vi "HRTF-Devices Dialog (TDT).vi"(1 "Path":path) -> (8 "Canceled?":bool)   [LabVIEW 2015]
uses:
  Utility VIs/Controls/KTable/KTable.xctl
  Typedefs/HRTF-Hardware Config (TDT).ctl
  PXI DAQ VIs/TDT VIs/Typedefs/TDT-Output source.ctl
  PXI DAQ VIs/TDT VIs/Typedefs/TDT-Device ID.ctl
  PXI DAQ VIs/TDT VIs/TDT-Globals.vi
panel:
  in  "InputTable":u16(xcontrol)
  in  "OutputTable":u16(xcontrol)
  out "Image":enum32{"None", "RX6", "RZ5", "RZ6"}(tab)
  in  "Run on":u16(ring) items=["RX6", "RZ5", "RZ6"]
  out "exit signal":bool
  in  "Cancel":bool
  in  "OK":bool
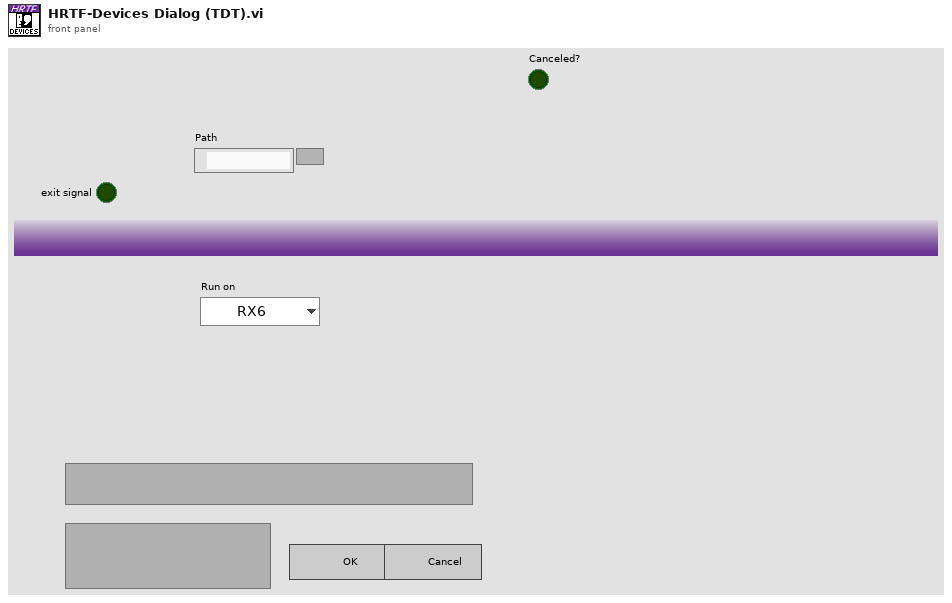
[diagram p1: front panel]
types:
  T1 = typedef "HRTF-Hardware Config (TDT).ctl" = cluster{"Output":T2, "Speaker":cluster{"Channel":i32, "Primary mux":i32, "Secondary mux":i32}, "Right mic":i32, "Left mic":i32}
  T2 = typedef "TDT-Output source.ctl" = cluster{"Device":T3, "Num":i32}
  T3 = typedef "TDT-Device ID.ctl" = enum16{"None", "PA5", "RP2", "RL2", "RA16", "RV8", "RX5", "RX6", "RX7", "RX8", "RZ2", "RZ5", "RZ6"}
  T4 = cluster{string, "Channel":i32, "Primary mux":i32, "Secondary mux":i32}
  T5 = cluster{string, "Channel":i32, "Primary mux":i32, "Secondary mux":i32}[]
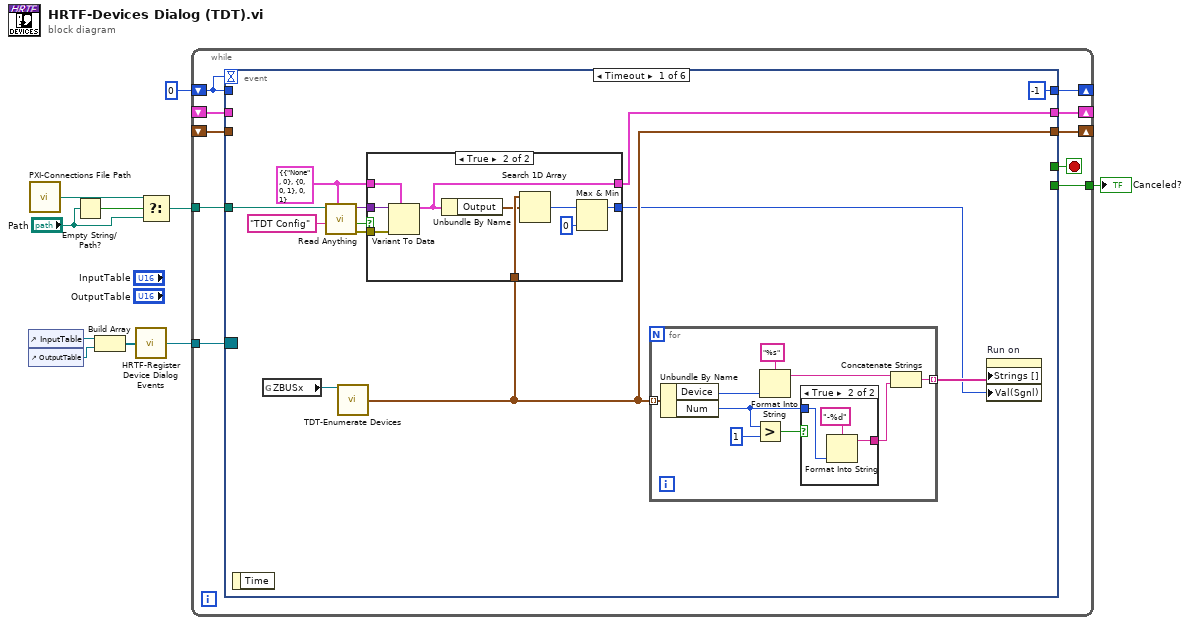
[diagram p0: block diagram]
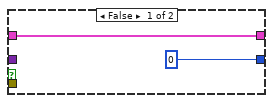
[diagram p2: hidden frame]
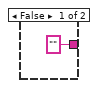
[diagram p3: hidden frame]
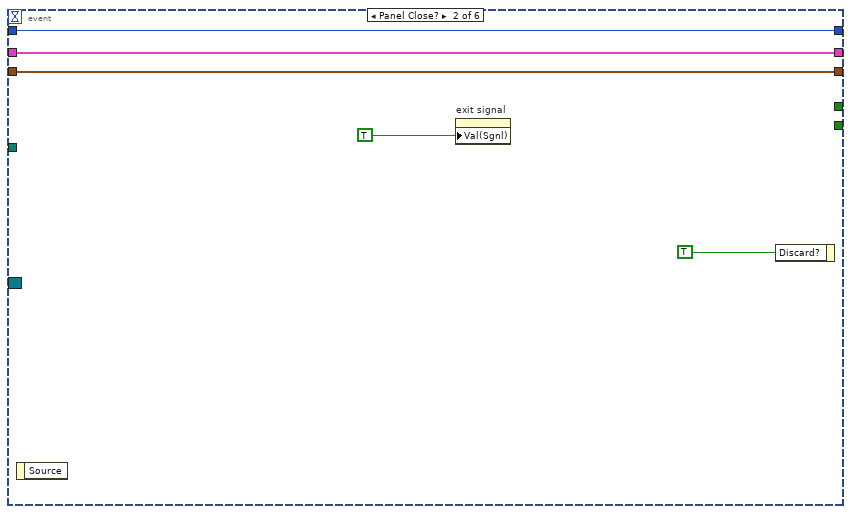
[diagram p4: hidden frame]
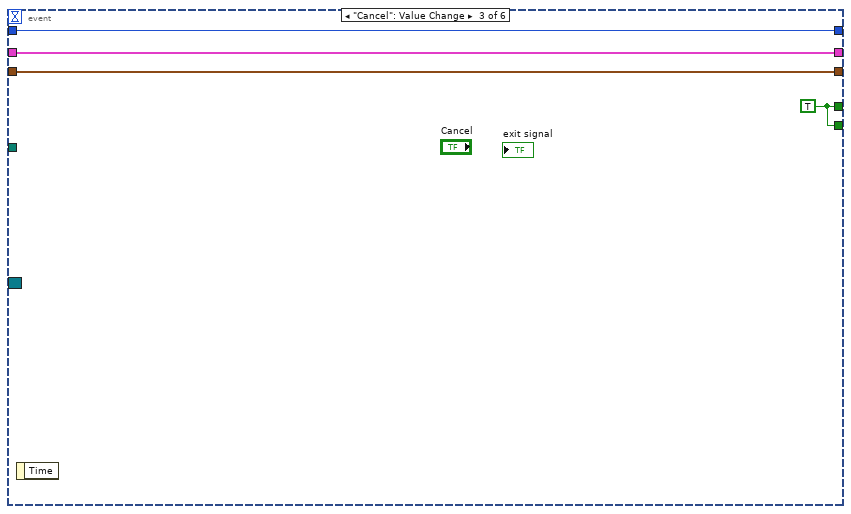
[diagram p5: hidden frame]
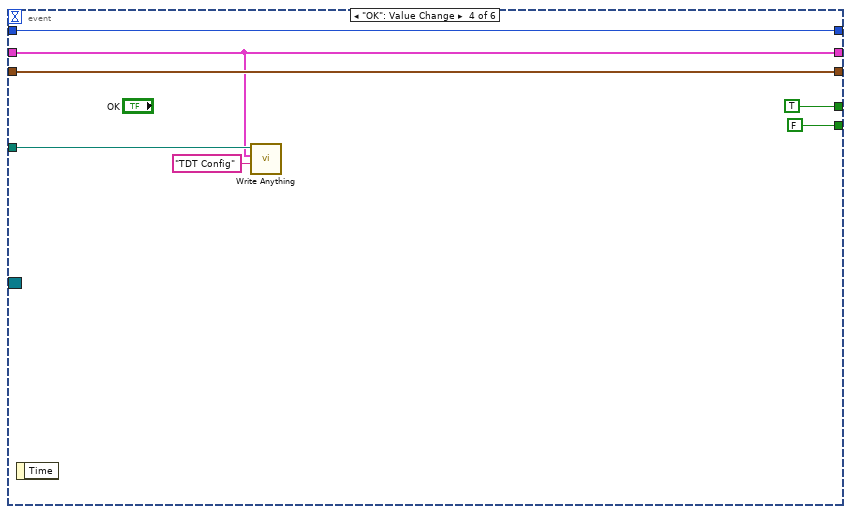
[diagram p6: hidden frame]
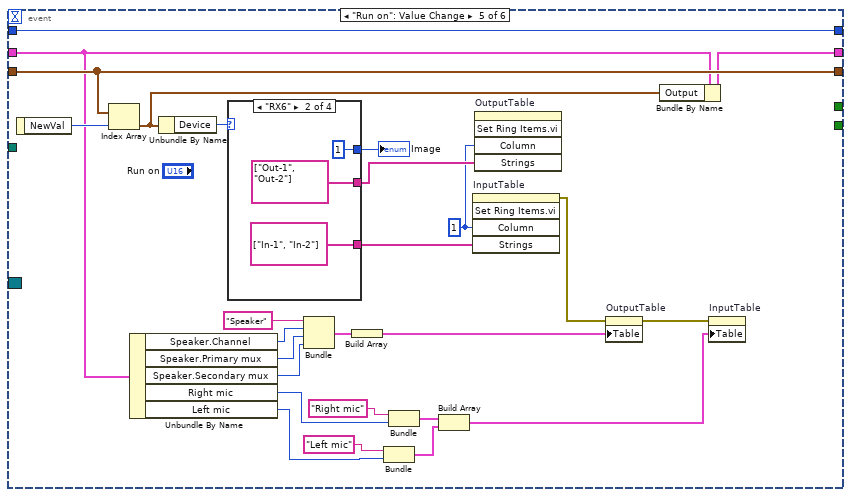
[diagram p7: hidden frame]
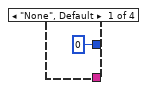
[diagram p8: hidden frame]
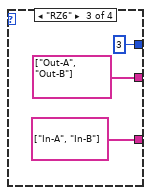
[diagram p9: hidden frame]
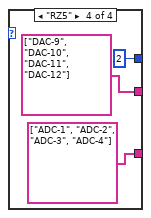
[diagram p10: hidden frame]
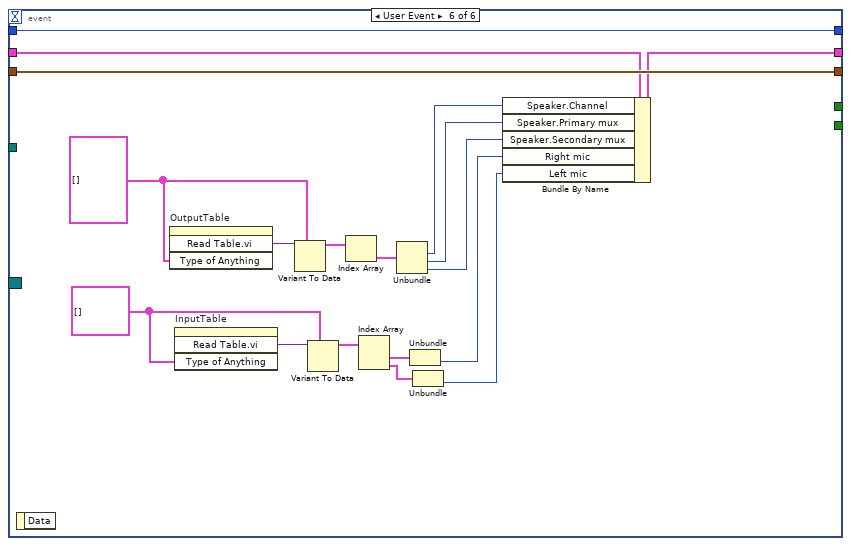
[diagram p11: hidden frame]
diagram:
  n1 = control-ref of="InputTable"() -> (w4:refnum<vi>)
  n2 = control-ref of="OutputTable"() -> (w3:refnum<vi>)
  n3 = call "PXI-Connections File Path.vi"() -> ("Path"=w7:path)  [unwired: 1 in]
  n4 = Empty String/Path?(string/path="Path") -> (empty?=w8:bool)
  n5 = Build Array(w4, w3) -> (w2:refnum<vi>[])
  n6 = call "HRTF-Register Device Dialog Events.vi"("Refs"=w2) -> ("Event Registration Refnum"=w1:refnum<event-registration>)  [unwired: 13 in, 1 out]
  n7 = Select(t=w7, s=w8, f="Path") -> (s? t:f=w5:path)
  n8 = while {
    shift-right: [w20] -> _
    shift-left: 0 -> [w17]
    tunnel: [w18] -> w9
    shift-right: [w16] -> _
    shift-left: _ -> [w15]
    tunnel: w5 -> [w14]
    shift-right: [w13] -> _
    shift-left: _ -> [w12]
    tunnel: w1 -> [w11]
    stop <- w19 stop-if-true
    n9 = event shown="[0] Timeout" {
      selector: w11 -> [_ _ _ _ _ _]
      dyn-events: _ -> [_ _ _ _ _ _]
      timeout: w17 -> [_ _ _ _ _ _]
      tunnel: [-1 w61 w64 w70 w98 w126] -> w20
      tunnel: [_ _ w65 TRUE _ _] -> w19
      tunnel: [_ _ w65 FALSE _ _] -> w18
      tunnel: w17 -> [_ w61 w64 w70 w98 w126]
      tunnel: [w25 w58 w63 w69 w97 w125] -> w16
      tunnel: w15 -> [_ w58 w63 w69 w97 w125]
      tunnel: w14 -> [w30 _ _ w68 _ _]
      tunnel: [w21 w57 w62 w67 w74 w119] -> w13
      tunnel: w12 -> [_ w57 w62 w67 w90 w124]
      event Timeout {
        w22 = T1 {"Output"={"Device"=enum."None", "Num"=0}, "Speaker"={"Channel"=0, "Primary mux"=0, "Secondary mux"=1}, "Right mic"=0, "Left mic"=1} ("TDT")
        n10 = event-data() -> ()  [unwired: 1 in, 1 out]
        n11 = global read "TDT-Globals.vi" "ZBUSx"() -> (w23:refnum<k7>)
        n12 = call "Read Anything.vi"("Type of Anything"=w22, "Section Name (Name of \"Type of Anything\")"="TDT Config" ("Section Name (Name of \"Type of Anything\")"), "Path (dialog)"=w30) -> ("Error Out"=w28:errorcluster, "Found?"=w27:bool, "Anything"=w26:variant)  [unwired: 6 in]
        n13 = call "TDT-Enumerate Devices.vi"("ZBUSx In"=w23) -> ("Devices"=w25:T2[])  [unwired: 12 in, 2 out]
        n14 = case shown="True" w27 {
          tunnel: w28 -> [_ w43]
          tunnel: w26 -> [_ w42]
          tunnel: w22 -> [w33 w41]
          tunnel: w25 -> [_ w38]
          tunnel: [0 w37] -> w24
          tunnel: [w33 w35] -> w21
          frame False {
          }
          frame True {
            n15 = Variant To Data(error in=w43, type=w41, Variant=w42) -> (data=w35:T1)  [unwired: 1 out]
            n16 = Unbundle By Name(w35) -> ("Output"=w36:T2)
            n17 = Search 1D Array(1D array=w38, element=w36) -> (index of element=w39:i32)  [unwired: 1 in]
            n18 = Max & Min(x=w39, y=0) -> (max(x,y)=w37:i32)  [unwired: 1 out]
          }
        }
        n19 = for {
          tunnel: w25 -> [w52] mode=indexing
          tunnel: [w46] -> w31 mode=indexing
          n20 = Unbundle By Name(w52) -> ("Device"=w44:T3, "Num"=w47:i32)
          n21 = Greater?(x=w47, y=1) -> (0:w48:bool)
          n22 = Format Into String(format string="%s", w44) -> (resulting string=w50:string)  [unwired: 2 in, 1 out]
          n23 = case shown="True" w48 {
            tunnel: w47 -> [_ w55]
            tunnel: ["" w54] -> w45
            frame False {
            }
            frame True {
              n24 = Format Into String(format string="-%d", w55) -> (resulting string=w54:string)  [unwired: 2 in, 1 out]
            }
          }
          n25 = Concatenate Strings(w50, w45) -> (w46:string)
        }
        n26 = property on="Run on" class="Ring (strict)"("Strings []"=w31, "Val(Sgnl)"=w24) -> ()  [unwired: 2 in, 2 out]
      }
      event Panel Close? {
        n27 = event-data() -> ()  [unwired: 1 in, 1 out]
        n28 = property on="exit signal" class="Bool (strict)"("Val(Sgnl)"=TRUE ("Value (Signaling)")) -> ()  [unwired: 2 in, 2 out]
        n29 = event-data("Discard?"=TRUE) -> ()  [unwired: 1 in, 1 out]
      }
      event "Cancel": Value Change {
        w65 = TRUE
        n30 = event-data() -> ()  [unwired: 1 in, 1 out]
      }
      event "OK": Value Change {
        n31 = event-data() -> ()  [unwired: 1 in, 1 out]
        n32 = call "Write Anything.vi"("Section Name (Name of \"Anything\")"="TDT Config" ("Section Name (Name of \"Anything\")"), "Anything"=w67, "Path (dialog)"=w68) -> ()  [unwired: 7 in, 2 out]
      }
      event "Run on": Value Change {
        w91 = 1
        n33 = event-data() -> ("NewVal"=w96:u16)  [unwired: 1 in]
        n34 = Index Array(array=w97, index=w96) -> (element=w73:T2)
        n35 = Unbundle By Name(w90) -> ("Speaker.Channel"=w88:i32, "Speaker.Primary mux"=w87:i32, "Speaker.Secondary mux"=w86:i32, "Right mic"=w82:i32, "Left mic"=w79:i32)
        n36 = Unbundle By Name(w73) -> ("Device"=w94:T3)
        n37 = case shown="\"RX6\"" w94 {
          tunnel: [0 1 3 2] -> w95
          tunnel: [_ string[] ["Out-1", "Out-2"] string[] ["Out-A", "Out-B"] string[] ["DAC-9", "DAC-10", "DAC-11", "DAC-12"]] -> w92
          tunnel: [_ string[] ["In-1", "In-2"] string[] ["In-A", "In-B"] string[] ["ADC-1", "ADC-2", "ADC-3", "ADC-4"]] -> w93
          frame "None", Default {
          }
          frame "RX6" {
          }
          frame "RZ6" {
          }
          frame "RZ5" {
          }
        }
        "Image" <- w95
        n38 = Bundle("Speaker", "Channel"=w88, "Primary mux"=w87, "Secondary mux"=w86) -> (w85:T4)  [unwired: 1 in]
        n39 = Build Array(w85) -> (w84:T5)
        n40 = Bundle("Left mic", "Left mic"=w79) -> (w77:cluster{string, "Left mic":i32})  [unwired: 1 in]
        n41 = Bundle("Right mic", "Right mic"=w82) -> (w78:cluster{string, "Right mic":i32})  [unwired: 1 in]
        n42 = Build Array(w78, w77) -> (w76:cluster{string, "Left mic":i32}[])
        n43 = invoke on="InputTable" class="KTable (strict)" method="Set Ring Items.vi"("Column"=w91, "Strings"=w93) -> (error out=w83:errorcluster)  [unwired: 3 in, 4 out]
        n44 = invoke on="OutputTable" class="KTable (strict)" method="Set Ring Items.vi"("Column"=w91, "Strings"=w92) -> ()  [unwired: 3 in, 5 out]
        n45 = property on="OutputTable" class="KTable (strict)"(error in=w83, "Table"=w84) -> (error out=w75:errorcluster)  [unwired: 1 in, 1 out]
        n46 = Bundle By Name(cluster=w90, "Output"=w73) -> (w74:T1)
        n47 = property on="InputTable" class="KTable (strict)"(error in=w75, "Table"=w76) -> ()  [unwired: 1 in, 2 out]
      }
      event User Event {
        w112 = cluster{string, i32}[] []
        w122 = cluster{string, i32, i32, i32}[] []
        n48 = event-data() -> ()  [unwired: 1 in, 1 out]
        n49 = invoke on="OutputTable" class="KTable (strict)" method="Read Table.vi"("Type of Anything"=w122) -> ("Read Table.vi"=w123:variant)  [unwired: 3 in, 3 out]
        n50 = invoke on="InputTable" class="KTable (strict)" method="Read Table.vi"("Type of Anything"=w112) -> ("Read Table.vi"=w113:variant)  [unwired: 3 in, 3 out]
        n51 = Variant To Data(type=w122, Variant=w123) -> (data=w121:cluster{string, i32, i32, i32}[])  [unwired: 1 in, 1 out]
        n52 = Variant To Data(type=w112, Variant=w113) -> (data=w115:cluster{string, i32}[])  [unwired: 1 in, 1 out]
        n53 = Index Array(array=w121) -> (element=w120:cluster{string, i32, i32, i32})  [unwired: 1 in]
        n54 = Index Array(array=w115) -> (element #1=w114:cluster{string, i32}, element #2=w111:cluster{string, i32})  [unwired: 2 in]
        n55 = Unbundle(w120) -> (w118:i32, w117:i32, w116:i32)  [unwired: 1 out]
        n56 = Unbundle(w114) -> (w110:i32)  [unwired: 1 out]
        n57 = Unbundle(w111) -> (w109:i32)  [unwired: 1 out]
        n58 = Bundle By Name(cluster=w124, "Speaker.Channel"=w118, "Speaker.Primary mux"=w117, "Speaker.Secondary mux"=w116, "Right mic"=w110, "Left mic"=w109) -> (w119:T1)
      }
    }
  }
  "Canceled?" <- w9
